vi "选择功能.vi"(9 "错误输入（无错误）":errorcluster, 10 "功能":string, 11 "按钮":refnum<vi>) -> (0 "方向":string, 1 "错误输出":errorcluster, 2 "正向":bool, 3 "功能输出":string)   [LabVIEW 2021]
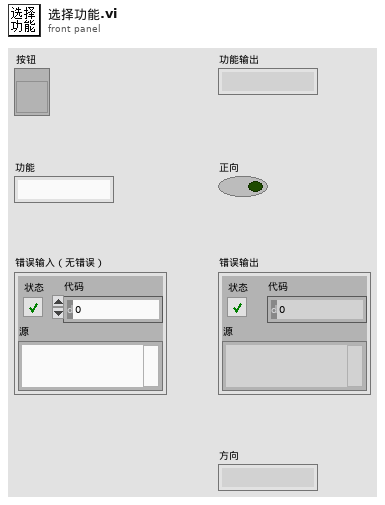
[diagram p1: front panel]
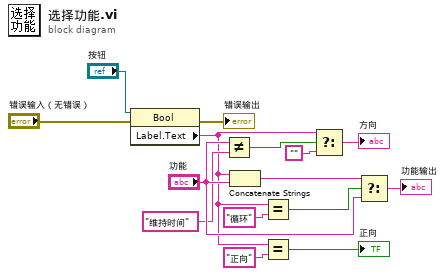
[diagram p0: block diagram]
diagram:
  n1 = property class="Bool"(reference="按钮", error in="错误输入（无错误）") -> (error out=→"错误输出":errorcluster, "Label.Text"=w2:string)  [unwired: 1 out]
  n2 = Not Equal?(x="功能", y="维持时间") -> (x != y?=w4:bool)
  n3 = Concatenate Strings(w2, "功能") -> (w12:string)
  n4 = Equal?(x=w2, y="循环") -> (x = y?=w11:bool)
  n5 = Equal?(x=w2, y="正向" ("x")) -> (x = y?=→"正向":bool)
  n6 = Select(t=w2, s=w4, f="") -> (s? t:f=→"方向":string)
  n7 = Select(t=w12, s=w11, f="功能") -> (s? t:f=→"功能输出":string)
